vi "Start Measurement.vi"(8 "error in (no error)":errorcluster, 11 "KeithleyMeter in":refnum<class "KeithleyMeter.lvclass">) -> (0 "error out":errorcluster, 3 "KeithleyMeter out":refnum<class "KeithleyMeter.lvclass">)   [LabVIEW 2015, in "KeithleyMeter.lvclass"]
uses:
  KeithleyMeter.lvclass
  Keithley Meter Parameters.ctl
  KeithleyMeter Function.ctl
  Instrument/Read VISA Resource.vi
  OO Devices/Device/Read Controls Snapshot.vi
  Instrument/Write VISA Resource.vi
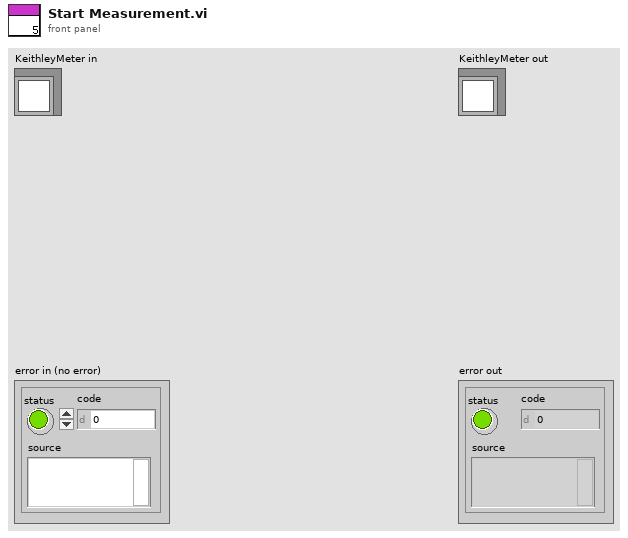
[diagram p1: front panel]
types:
  T1 = typedef "Keithley Meter Parameters.ctl" = cluster{"Range (-1: auto)":dbl, "Integration Time (NPLCs)":dbl, "Function":T2, "W Offset comp":bool, "4-wire W":bool, "Scale":dbl, "Offset":dbl}
  T2 = typedef "KeithleyMeter Function.ctl" = enum16{"VOLTAGE", "CURRENT", "RESISTANCE"}
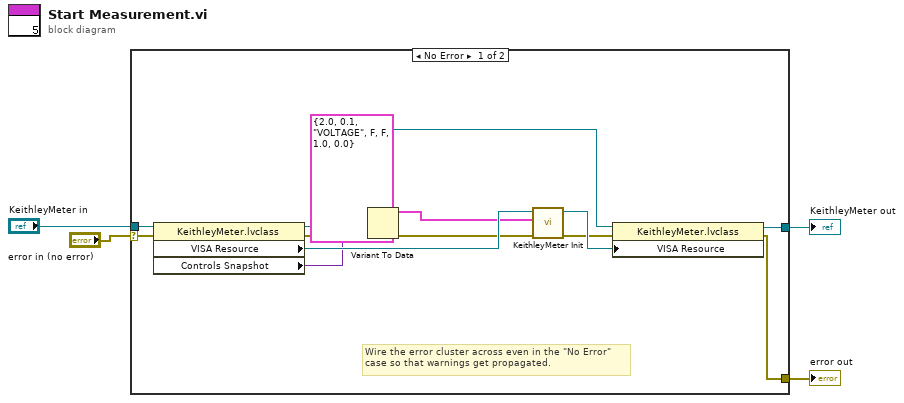
[diagram p0: block diagram]
diagram:
  n1 = case shown="No Error" "error in (no error)" {
    selector: "error in (no error)" -> [w16 w19]
    tunnel: [w6 w19] -> w3
    tunnel: [w7 w18] -> w1
    tunnel: "KeithleyMeter in" -> [w17 w18]
    frame No Error {
      # "Wire the error cluster across even in the \"No Error\"\ncase so that warnings get propagated."
      n2 = property class="KeithleyMeter.lvclass"(reference=w17, error in=w16) -> (reference out=w8:refnum<class "KeithleyMeter.lvclass">, error out=w13:errorcluster, "VISA Resource"=w14:refnum<visa-resource-name>, "Controls Snapshot"=w12:variant)
      n3 = Variant To Data(error in=w13, type=T1 {"Range (-1: auto)"=2.0, "Integration Time (NPLCs)"=0.1, "Function"=enum."VOLTAGE", "W Offset comp"=FALSE, "4-wire W"=FALSE, "Scale"=1.0, "Offset"=0.0} ("Parameters"), Variant=w12) -> (data=w5:T1, error out=w10:errorcluster)
      n4 = call "KeithleyMeter Init.vi"("Error In"=w10, "Parameters"=w5, "VISA resource name"=w14) -> ("Error Out"=w9:errorcluster, "VISA resource name out"=w15:refnum<visa-resource-name>)  [unwired: 7 in]
      n5 = property class="KeithleyMeter.lvclass"(reference=w8, error in=w9, "VISA Resource"=w15) -> (reference out=w7:refnum<class "KeithleyMeter.lvclass">, error out=w6:errorcluster)
    }
    frame Error {
    }
  }
  "error out" <- w3
  "KeithleyMeter out" <- w1
